vi "GPI-Load-Save settings.vi"() -> ()   [LabVIEW 2011]
doc: "This VI allows for the saving and loading of the configuration\nof the controls in this VI."
uses:
  Saved VI controls.ctl
panel:
  out "File data":T1(array[cluster])
  in  "Save settings of these VIs:":string[](array[string])=["Multi-mode acquisition.vi", "autofocus globals.vi", "stage step to next field.vi"]
  in  "stop":bool
  in  "Load Configuration":bool
  in  "Save Configuration":bool
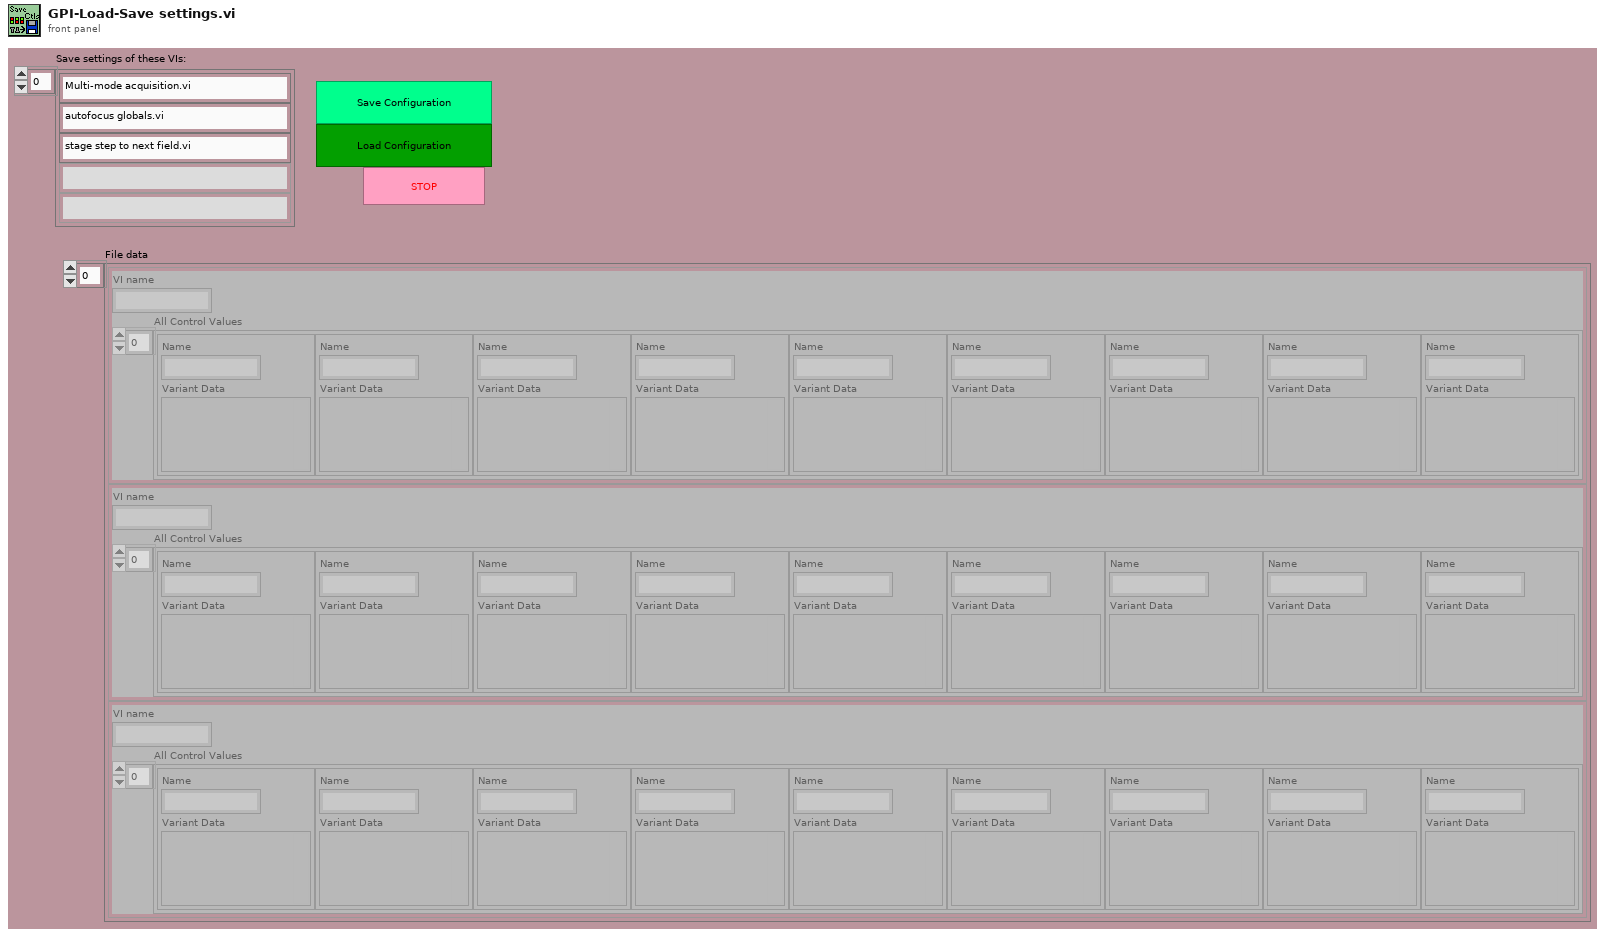
[diagram p1: front panel]
types:
  T1 = cluster{"VI name":string, "All Control Values":cluster{"Name":string, "Variant Data":variant}[]}[]
  T2 = typedef "Saved VI controls.ctl" = cluster{"VI name":string, "All Control Values":cluster{"Name":string, "Variant Data":variant}[]}
  T3 = enum16{"open", "open or create", "create or replace", "create", "open (read only)"}
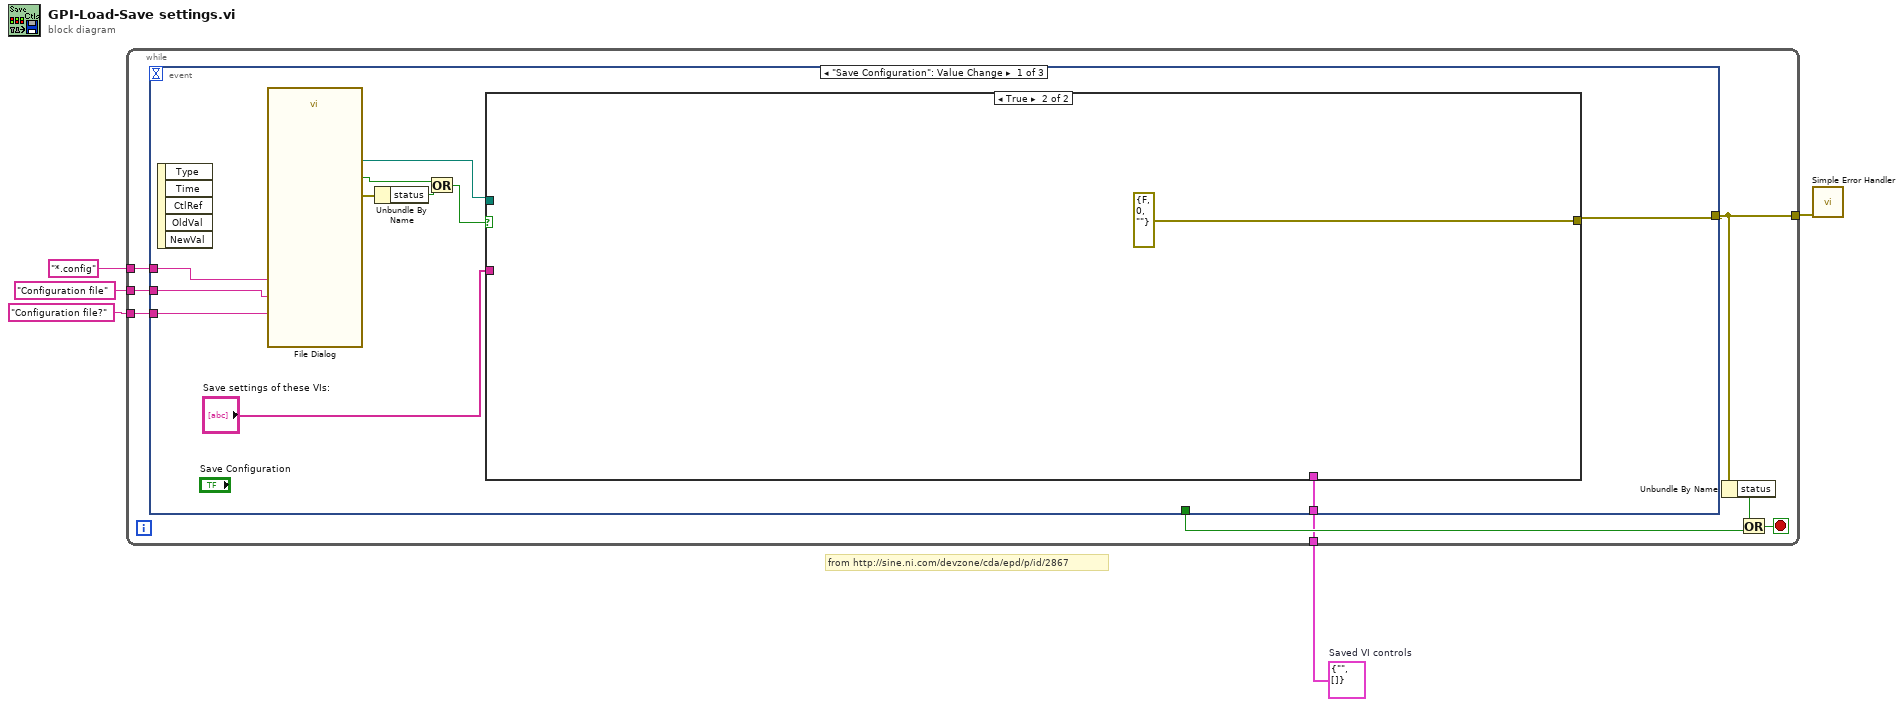
[diagram p0: block diagram]
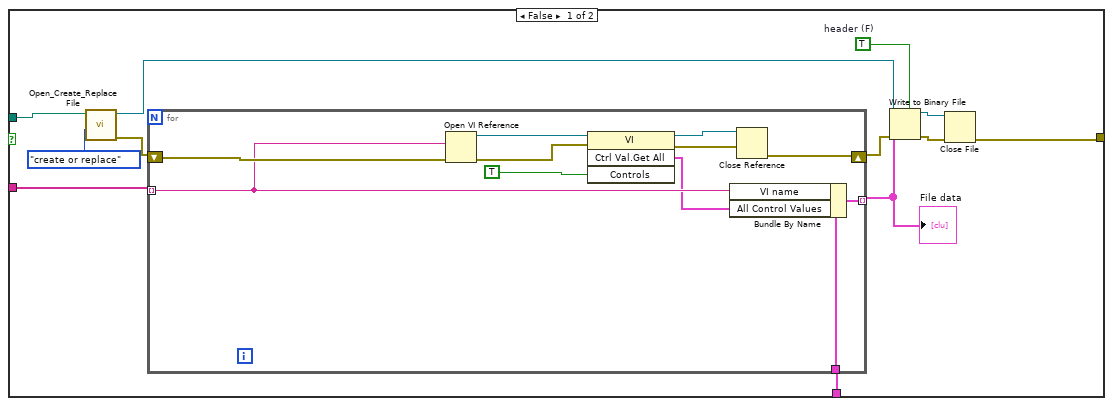
[diagram p2: hidden frame]
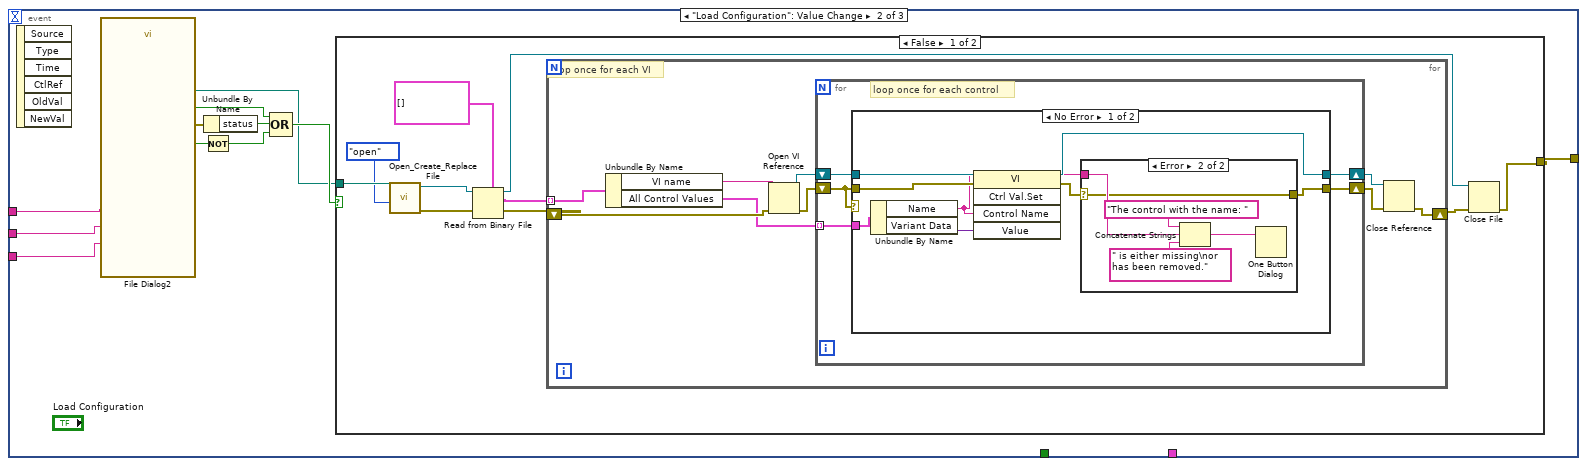
[diagram p3: hidden frame]
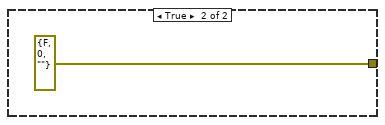
[diagram p6: hidden frame]
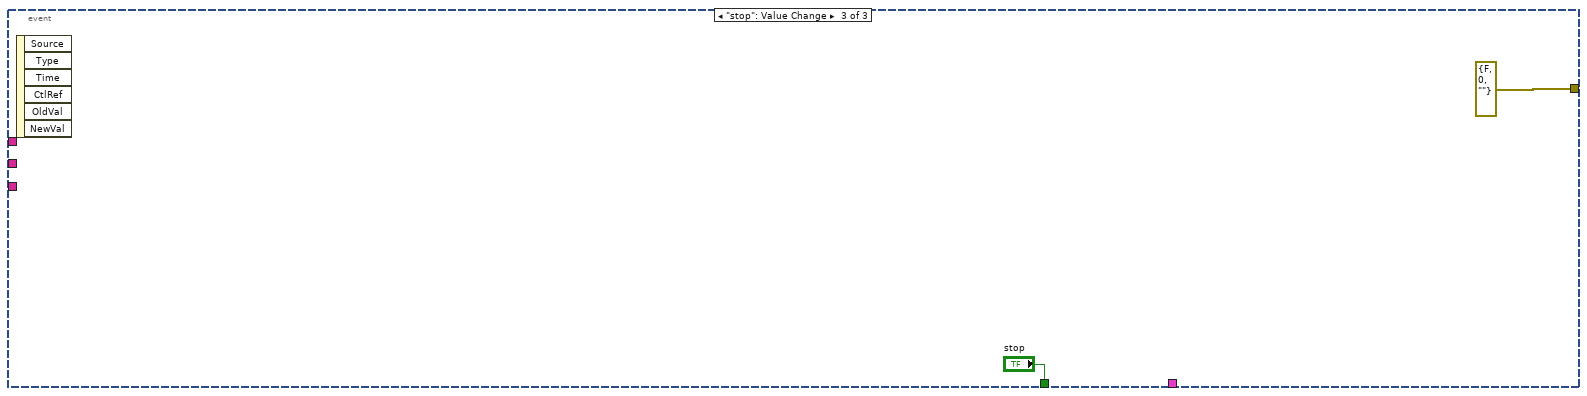
[diagram p7: hidden frame]
diagram:
  w4 = T2 {"VI name"="", "All Control Values"=[]}  # Saved VI controls
  # "from http://sine.ni.com/devzone/cda/epd/p/id/2867"
  n1 = while {
    tunnel: [w10] -> w5
    tunnel: w4 -> [w9]
    tunnel: "*.config" ("default name") -> [w8]
    tunnel: "Configuration file?" ("prompt") -> [w7]
    tunnel: "Configuration file" ("prompt") -> [w6]
    stop <- w12 stop-if-true
    n2 = event shown="[0] \"Save Configuration\": Value Change" {
      selector: _ -> [_ _ _]
      dyn-events: _ -> [_ _ _]
      timeout: _ -> [_ _ _]
      tunnel: [_ _ "stop"] -> w13
      tunnel: [w23 w59 errorcluster {"status"=FALSE, "code"=0, "source"=""} ("error out")] -> w10
      tunnel: w9 -> [w21 _ _]
      tunnel: w8 -> [w15 w58 _]
      tunnel: w7 -> [w17 w57 _]
      tunnel: w6 -> [w14 w49 _]
      event "Save Configuration": Value Change {
        n3 = event-data() -> ()  [unwired: 6 out]
        n4 = call "File Dialog"("prompt"=w17, "pattern (all files)"=w15, "pattern label"=w14) -> ("selected path"=w24:path, "cancelled"=w19:bool, "error out"=w16:errorcluster)  [unwired: 9 in, 1 out]
        n5 = Unbundle By Name(w16) -> ("status"=w20:bool)
        n6 = Or(x=w19, y=w20) -> (x .or. y?=w18:bool)
        n7 = case shown="True" w18 {
          tunnel: w24 -> [w34 _]
          tunnel: [w28 errorcluster {"status"=FALSE, "code"=0, "source"=""} ("error out")] -> w23
          tunnel: "Save settings of these VIs:" -> [w36 _]
          tunnel: w21 -> [w25 _]
          frame False {
            w26 = TRUE  # header (F)
            n8 = call <vilib>:"Open_Create_Replace File.vi"("function (open:0)"=T3."create or replace", "file path"=w34) -> ("error out"=w33:errorcluster, "refnum"=w32:refnum<file>)  [unwired: 4 in, 4 out]
            n9 = for {
              tunnel: w36 -> [w43] mode=indexing
              shift-right: [w40] -> w31
              shift-left: w33 -> [w46]
              tunnel: [w39] -> w27 mode=indexing
              tunnel: w25 -> [w38]
              n10 = Open VI Reference(vi path=w43, error in (no error)=w46) -> (vi reference=w45:refnum<vi>, error out=w44:errorcluster)  [unwired: 4 out]
              n11 = invoke on="Invoke Node" class="VI" method="Ctrl Val.Get All"(reference=w45, error in=w44, "Controls"=TRUE ("controls")) -> (reference out=w41:refnum<vi>, error out=w42:errorcluster, "Get All Control Values Variant"=w37:cluster{"Name":string, "Variant Data":variant}[])  [unwired: 1 in, 1 out]
              n12 = Bundle By Name(cluster=w38, "VI name"=w43, "All Control Values"=w37) -> (w39:T2)
              n13 = Close Reference(reference=w41, error in (no error)=w42) -> (error out=w40:errorcluster)
            }
            "File data" <- w27
            n14 = Write to Binary File ("Write File")(file (use dialog)=w32, data=w27, error in=w31, 5:w26) -> (refnum out=w29:refnum<file>, error out=w30:errorcluster)  [unwired: 3 out]
            n15 = Close File(refnum=w29, error in=w30) -> (error out=w28:errorcluster)  [unwired: 1 out]
          }
          frame True {
          }
        }
      }
      event "Load Configuration": Value Change {
        n16 = event-data() -> ()  [unwired: 7 out]
        n17 = call "File Dialog2"("prompt"=w57, "pattern (all files)"=w58, "pattern label"=w49) -> ("selected path"=w50:path, "exists"=w52:bool, "cancelled"=w54:bool, "error out"=w56:errorcluster)  [unwired: 9 in]
        n18 = Not(x=w52) -> (.not. x?=w53:bool)
        n19 = Unbundle By Name(w56) -> ("status"=w55:bool)
        n20 = Compound Arithmetic op=OR(w54, w55, w53) -> (w51:bool)
        n21 = case shown="False" w51 {
          tunnel: w50 -> [w68 _]
          tunnel: [w65 errorcluster {"status"=FALSE, "code"=0, "source"=""} ("error out")] -> w59
          frame False {
            n22 = call <vilib>:"Open_Create_Replace File.vi"("function (open:0)"=T3."open", "file path"=w68) -> ("error out"=w64:errorcluster, "refnum"=w63:refnum<file>)  [unwired: 4 in, 4 out]
            n23 = Read from Binary File ("Read File")(5:T2[] [], 11:w63) -> (2:w60:T2[], 3:w62:refnum<file>)  [unwired: 1 in, 5 out]
            n24 = for {
              shift-right: [w70] -> w66
              shift-left: w64 -> [w76]
              tunnel: w60 -> [w69] mode=indexing
              # "loop once for each VI"
              n25 = Unbundle By Name(w69) -> ("VI name"=w77:string, "All Control Values"=w75:cluster{"Name":string, "Variant Data":variant}[])
              n26 = Open VI Reference(vi path=w77, error in (no error)=w76) -> (vi reference=w73:refnum<vi>, error out=w74:errorcluster)  [unwired: 4 out]
              n27 = for {
                tunnel: w75 -> [w82] mode=indexing
                shift-right: [w79] -> w72
                shift-left: w73 -> [w80]
                shift-right: [w81] -> w71
                shift-left: w74 -> [w78]
                # "loop once for each control"
                n28 = case shown="No Error" w78 {
                  tunnel: w82 -> [w89 _]
                  tunnel: w78 -> [w88 w97]
                  tunnel: [w86 w97] -> w81
                  tunnel: w80 -> [w85 w98]
                  tunnel: [w84 w98] -> w79
                  frame No Error {
                    n29 = Unbundle By Name(w89) -> ("Name"=w83:string, "Variant Data"=w90:variant)
                    n30 = invoke on="Invoke Node" class="VI" method="Ctrl Val.Set"(reference=w85, error in=w88, "Control Name"=w83, "Value"=w90) -> (reference out=w84:refnum<vi>, error out=w87:errorcluster)  [unwired: 1 in, 3 out]
                    n31 = case shown="Error" w87 {
                      selector: w87 -> [w91 w92]
                      tunnel: w83 -> [_ w95]
                      tunnel: [w91 w92] -> w86
                      frame No Error {
                      }
                      frame Error {
                        n32 = Concatenate Strings("The control with the name: " ("string"), w95, " is either missing\nor has been removed." ("string")) -> (w93:string)
                        n33 = One Button Dialog(message=w93) -> ()  [unwired: 2 out]
                      }
                    }
                  }
                  frame Error {
                  }
                }
              }
              n34 = Close Reference(reference=w72, error in (no error)=w71) -> (error out=w70:errorcluster)
            }
            n35 = Close File(refnum=w62, error in=w66) -> (error out=w65:errorcluster)  [unwired: 1 out]
          }
          frame True {
          }
        }
      }
      event "stop": Value Change {
        n36 = event-data() -> ()  [unwired: 7 out]
      }
    }
    n37 = Unbundle By Name(w10) -> ("status"=w11:bool)
    n38 = Or(x=w11, y=w13) -> (x .or. y?=w12:bool)
  }
  n39 = call <vilib>:"Simple Error Handler.vi"("error in (no error)"=w5) -> ()  [unwired: 1 in, 8 out]
